vi "5-4GrafiklerveFitting.vi"() -> ()   [LabVIEW 2024]
uses:
  <vilib>/Analysis/NI_AALPro.lvlib
panel:
  out "slope 2":dbl
  out "residue 2":dbl
  out "XY Graph 3":cluster{"x":dbl[], "Best Linear Fit":dbl[]}[](graph)
  in  "y 2":dbl[](array[numeric])
  in  "x 2":dbl[](array[numeric])
  out "residue":dbl
  out "slope":dbl
  out "XY Graph 2":cluster{"x":dbl[], "Best Linear Fit":dbl[]}[](graph)
  in  "y":dbl[](array[numeric])
  in  "x":dbl[](array[numeric])
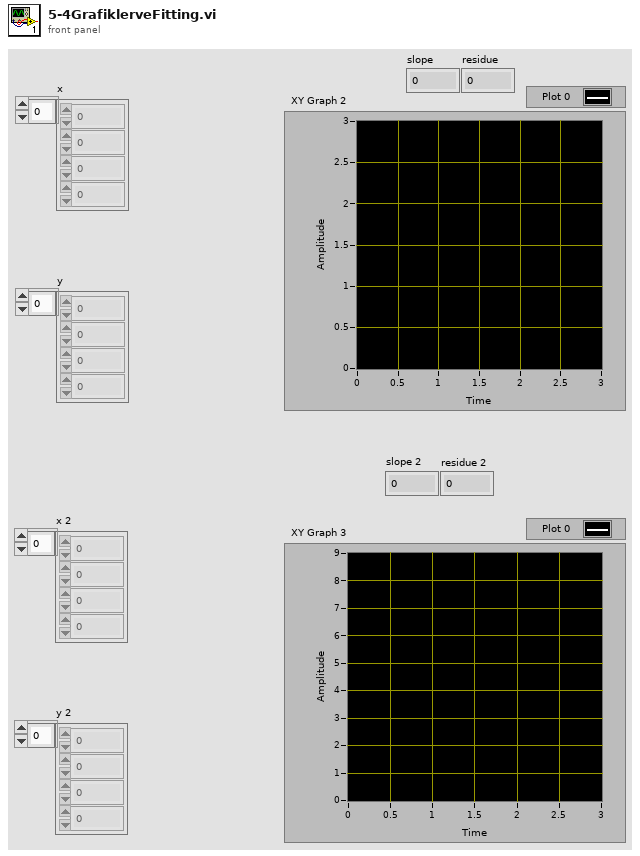
[diagram p1: front panel]
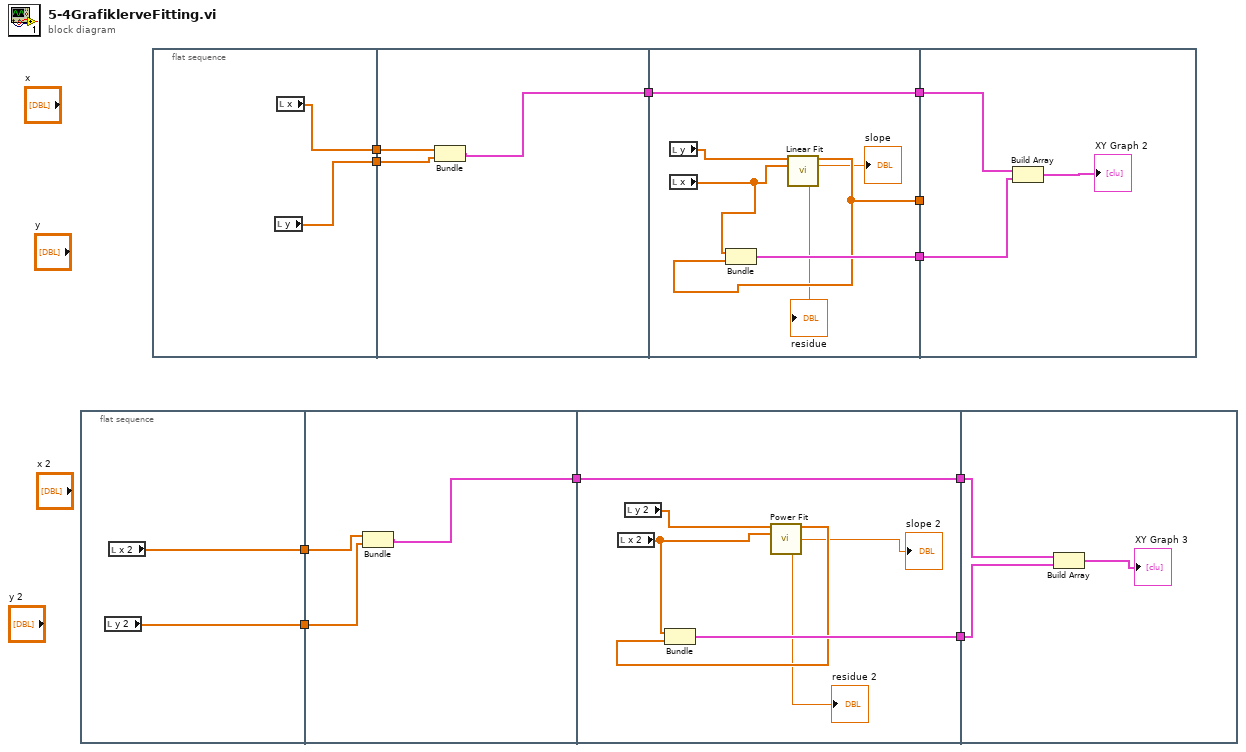
[diagram p0: block diagram]
diagram:
  n1 = flat-sequence {
    tunnel: [w13] -> w3
    tunnel: [w12] -> w2
    tunnel: [w16] -> w5
    tunnel: w3 -> [w15]
    tunnel: w2 -> [w14]
    tunnel: [w23] -> w4
    tunnel: w5 -> [w23]
    tunnel: [w22] -> w1
    tunnel: w4 -> [w26]
    tunnel: w1 -> [w24]
    frame #0 {
      n2 = local read "y 2"() -> (w13:dbl[])
      n3 = local read "x 2"() -> (w12:dbl[])
    }
    frame #1 {
      n4 = Bundle("x 2"=w14, "y 2"=w15) -> (w16:cluster{"x 2":dbl[], "y 2":dbl[]})  [unwired: 1 in]
    }
    frame #2 {
      n5 = local read "x 2"() -> (w19:dbl[])
      n6 = local read "y 2"() -> (w20:dbl[])
      n7 = call <vilib>:"Power Fit.vi"("Y"=w20, "X"=w19) -> ("Best Power Fit"=w21:dbl[], "power"=→"slope 2":dbl, "residue"=→"residue 2":dbl)  [unwired: 8 in, 3 out]
      n8 = Bundle("x 2"=w19, "Best Power Fit"=w21) -> (w22:cluster{"x 2":dbl[], "Best Power Fit":dbl[]})  [unwired: 1 in]
    }
    frame #3 {
      n9 = Build Array(w26, w24) -> (→"XY Graph 3":cluster{"x 2":dbl[], "Best Power Fit":dbl[]}[])
    }
  }
  n10 = flat-sequence {
    tunnel: [w28] -> w11
    tunnel: [w27] -> w10
    tunnel: w11 -> [w31]
    tunnel: w10 -> [w30]
    tunnel: [w29] -> w8
    tunnel: [w36] -> w9
    tunnel: w8 -> [w36]
    tunnel: [w35] -> w7
    tunnel: [w34] -> w6
    tunnel: w9 -> [w41]
    tunnel: w7 -> [w40]
    tunnel: w6 -> [_]
    frame #0 {
      n11 = local read "y"() -> (w27:dbl[])
      n12 = local read "x"() -> (w28:dbl[])
    }
    frame #1 {
      n13 = Bundle("x"=w31, "y"=w30) -> (w29:cluster{"x":dbl[], "y":dbl[]})  [unwired: 1 in]
    }
    frame #2 {
      n14 = local read "y"() -> (w38:dbl[])
      n15 = local read "x"() -> (w37:dbl[])
      n16 = call <vilib>:"Linear Fit.vi"("Y"=w38, "X"=w37) -> ("Best Linear Fit"=w34:dbl[], "slope"=→"slope":dbl, "residue"=→"residue":dbl)  [unwired: 9 in, 2 out]
      n17 = Bundle("x"=w37, "Best Linear Fit"=w34) -> (w35:cluster{"x":dbl[], "Best Linear Fit":dbl[]})  [unwired: 1 in]
    }
    frame #3 {
      n18 = Build Array(w41, w40) -> (→"XY Graph 2":cluster{"x":dbl[], "Best Linear Fit":dbl[]}[])
    }
  }
